vi "popup_(SubVI).vi"(11 "X":i32) -> (3 "?":string)   [LabVIEW 2020]
panel:
  in  "?":bool
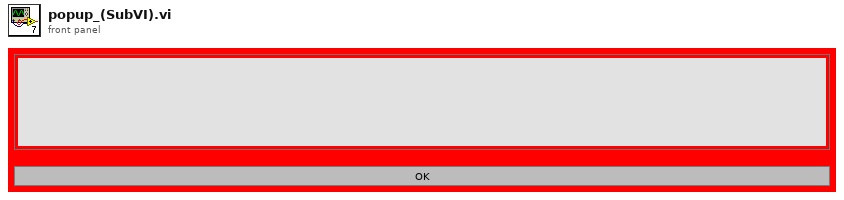
[diagram p1: front panel]
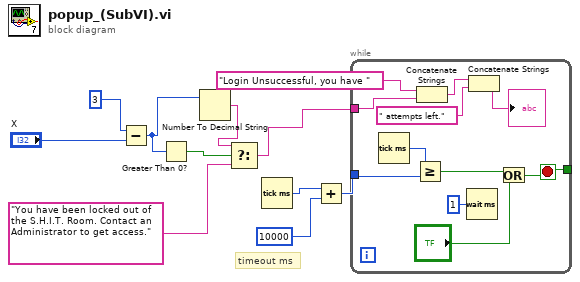
[diagram p0: block diagram]
diagram:
  # "timeout ms"
  n1 = Subtract(x=3, y="X") -> (x-y=w5:i32)
  n2 = Greater Than 0?(x=w5) -> (x > 0?=w4:bool)
  n3 = Number To Decimal String(number=w5) -> (decimal integer string=w1:string)  [unwired: 1 in]
  n4 = Select(t=w1, s=w4, f="You have been locked out of the S.H.I.T. Room. Contact an Administrator to get access.") -> (s? t:f=w2:string)
  n5 = Tick Count (ms)() -> (millisecond timer value=w6:u32)
  n6 = Add(x=w6, y=u32 10000) -> (x+y=w7:u32)
  n7 = while {
    tunnel: w7 -> [w20]
    tunnel: [w11] -> _
    tunnel: w2 -> [w18]
    stop <- w11 stop-if-true
    n8 = Tick Count (ms)() -> (millisecond timer value=w19:u32)
    n9 = Greater Or Equal?(x=w19, y=w20) -> (x >= y?=w13:bool)
    n10 = Concatenate Strings("Login Unsuccessful, you have " ("string"), w18) -> (w16:string)
    n11 = Wait (ms)(milliseconds to wait=u32 1 ("millisecond timer value")) -> ()  [unwired: 1 out]
    n12 = Concatenate Strings(w16, " attempts left." ("string")) -> (→"?":string)
    n13 = Or(x=w13, y="?") -> (x .or. y?=w11:bool)
  }
